vi "Remove Custom Device.vi"(8 "error in (no error)":errorcluster, 11 "Custom Device":refnum<k24>) -> (0 "error out":errorcluster)   [LabVIEW 2017, in "Switch Scripting.lvlib"]
uses:
  Switch Scripting.lvlib
  NationalInstruments.VeriStand.SystemDefinitionAPI
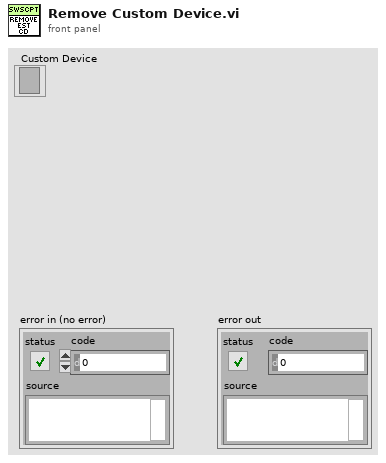
[diagram p1: front panel]
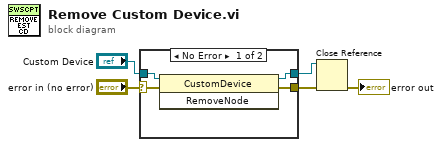
[diagram p0: block diagram]
diagram:
  n1 = case shown="No Error" "error in (no error)" {
    selector: "error in (no error)" -> [w8 w11]
    tunnel: "Custom Device" -> [w9 w10]
    tunnel: [w7 w10] -> w3
    tunnel: [w6 w11] -> w2
    frame No Error {
      n2 = invoke class="CustomDevice" method="RemoveNode"(reference=w9, error in=w8) -> (reference out=w7:refnum<k24>, error out=w6:errorcluster)  [unwired: 1 in, 1 out]
    }
    frame Error {
    }
  }
  n3 = Close Reference(reference=w3, error in (no error)=w2) -> (error out=→"error out":errorcluster)
